vi "Equip-Get Device (TDT).vi"(0 "Path In":path=path "C:/ProgramData/EPL/Tosca Defaults.ini", 7 "Default":T1={"Output"={"Device"=enum."RZ5", "Num"=0}, "Input"=enum."Front Panel"}, 11 "error in (no error)":errorcluster) -> (4 "Path Out":path=path "C:/ProgramData/EPL/Tosca Defaults.ini", 8 "TDT-Device Config":T1, 15 "error out":errorcluster)   [LabVIEW 2020]
uses:
  PXI DAQ VIs/TDT VIs/Typedefs/TDT-Device Config.ctl
  PXI DAQ VIs/TDT VIs/Typedefs/TDT-Output source.ctl
  PXI DAQ VIs/TDT VIs/Typedefs/TDT-Device ID.ctl
  PXI DAQ VIs/TDT VIs/Typedefs/TDT-Input source.ctl
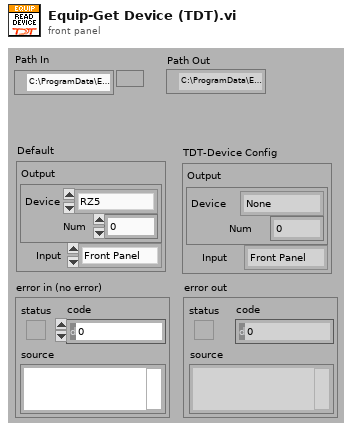
[diagram p1: front panel]
types:
  T1 = typedef "TDT-Device Config.ctl" = cluster{"Output":T2, "Input":T4}
  T2 = typedef "TDT-Output source.ctl" = cluster{"Device":T3, "Num":i32}
  T3 = typedef "TDT-Device ID.ctl" = enum16{"None", "PA5", "RP2", "RL2", "RA16", "RV8", "RX5", "RX6", "RX7", "RX8", "RZ2", "RZ5", "RZ6"}
  T4 = typedef "TDT-Input source.ctl" = enum16{"Front Panel", "RA4LI", "RA16LI"}
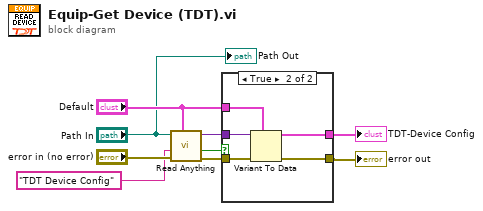
[diagram p0: block diagram]
diagram:
  n1 = call "Read Anything.vi"("Type of Anything"="Default", "Error In"="error in (no error)", "Section Name (Name of \"Type of Anything\")"="TDT Device Config" ("section"), "Path (dialog)"="Path In") -> ("Error Out"=w5:errorcluster, "Found?"=w7:bool, "Anything"=w6:variant)  [unwired: 5 in]
  n2 = case shown="True" w7 {
    tunnel: w6 -> [_ w15]
    tunnel: w5 -> [w10 w16]
    tunnel: "Default" -> [w11 w14]
    tunnel: [w11 w13] -> w3
    tunnel: [w10 w12] -> w2
    frame False {
    }
    frame True {
      n3 = Variant To Data(error in=w16, type=w14, Variant=w15) -> (data=w13:T1, error out=w12:errorcluster)
    }
  }
  "error out" <- w2
  "TDT-Device Config" <- w3
  "Path Out" <- "Path In"
